vi "create Timings.vi"(8 "error in (no error)":errorcluster, 10 "Parameters":u32[](array[numeric]), 11 "Surge in":refnum<class "Surge.lvclass">) -> (0 "error out":errorcluster, 1 "wait":i32[](array[numeric])=[0, 30000, 0, 0], 2 "timeout":u32[](array[numeric]), 3 "Surge out":refnum<class "Surge.lvclass">)   [LabVIEW 2013, in "Surge.lvclass"]
uses:
  Surge.lvclass
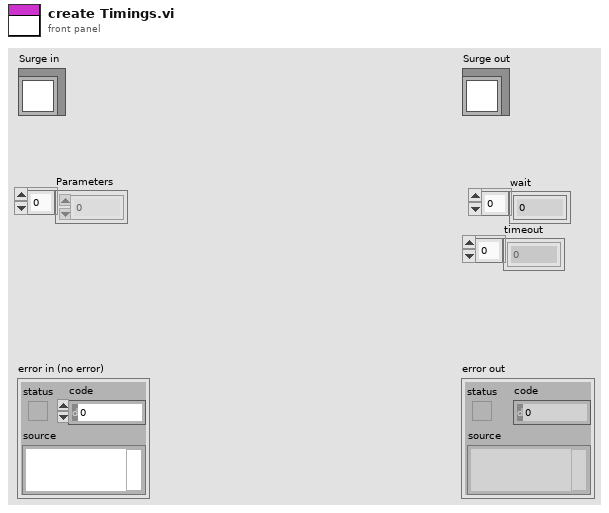
[diagram p1: front panel]
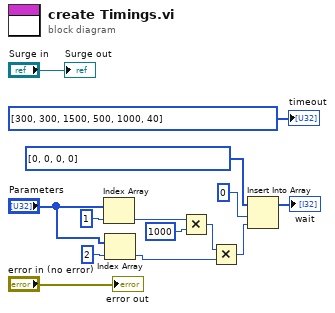
[diagram p0: block diagram]
diagram:
  n1 = Index Array(array="Parameters", index=1) -> (element=w13:u32)
  n2 = Index Array(array="Parameters", index=2) -> (element=w3:u32)
  n3 = Multiply(x=w13, y=u32 1000) -> (x*y=w2:u32)
  n4 = Multiply(x=w2, y=w3) -> (x*y=w1:u32)
  n5 = Insert Into Array(array=i32[] [0, 0, 0, 0] ("Timings"), index=0, new element=w1) -> (→"wait":i32[])
  "error out" <- "error in (no error)"
  "Surge out" <- "Surge in"
  "timeout" <- u32[] [300, 300, 1500, 500, 1000, 40] ("Timings")
